vi "Picture_Calculate_Origin.vi"(1 "Loaded Picture Width (in pixels)":i16, 2 "Y-Axis ratio (correction factor)":dbl, 3 "PictureBox.DrawAreaSize.Width":u32) -> (0 "Origin":T1)   [LabVIEW 2013]
uses:
  <vilib>/Utility/miscctls.llb/LVPointTypeDef.ctl
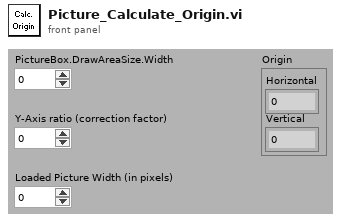
[diagram p1: front panel]
types:
  T1 = typedef "LVPointTypeDef.ctl" = cluster{"Horizontal":i16, "Vertical":i16}
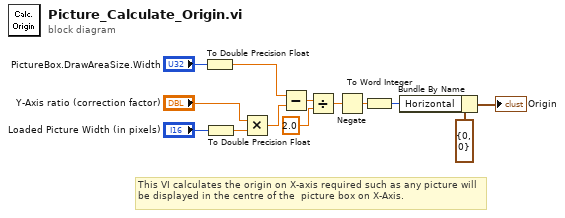
[diagram p0: block diagram]
diagram:
  # "This VI calculates the origin on X-axis required such as any picture will be displayed in the centre of the  picture box on X-Axis."
  n1 = To Double Precision Float(number="PictureBox.DrawAreaSize.Width") -> (double precision float=w3:dbl)
  n2 = To Double Precision Float(number="Loaded Picture Width (in pixels)") -> (double precision float=w4:dbl)
  n3 = Multiply(x="Y-Axis ratio (correction factor)", y=w4) -> (x*y=w1:dbl)
  n4 = Subtract(x=w3, y=w1) -> (x-y=w6:dbl)
  n5 = Divide(x=w6, y=2.0) -> (x/y=w8:dbl)
  n6 = Negate(x=w8) -> (-x=w11:dbl)
  n7 = To Word Integer(number=w11) -> (16bit integer=w13:i16)
  n8 = Bundle By Name(cluster=T1 {"Horizontal"=0, "Vertical"=0} ("Origin"), "Horizontal"=w13) -> (→"Origin":T1)
